vi "Plotmatrix Constructor.vi"(8 "error in (no error)":errorcluster, 9 "y matrix":dbl[][](array[numeric]), 10 "x matrix":dbl[][](array[numeric]), 11 "2D Plotmatrix Datatype.lvclass in":refnum<class "XY Plot Matrix Datatype.lvclass">) -> (0 "error out":errorcluster, 3 "2D Plotmatrix Datatype.lvclass out":refnum<class "XY Plot Matrix Datatype.lvclass">)   [LabVIEW 2020, in "XY Plot Matrix Datatype.lvclass"]
uses:
  <vilib>/Math Plots/2D Math Plots/XY Plot Matrix/XY Plot Matrix Datatype/XY Plot Matrix Datatype.lvclass
  <vilib>/Math Plots/2D Math Plots/XY Plot Matrix/XY Plot Matrix Datatype/XY Plot Matrix Datatype.lvclass/XY Plot Matrix Datatype.ctl
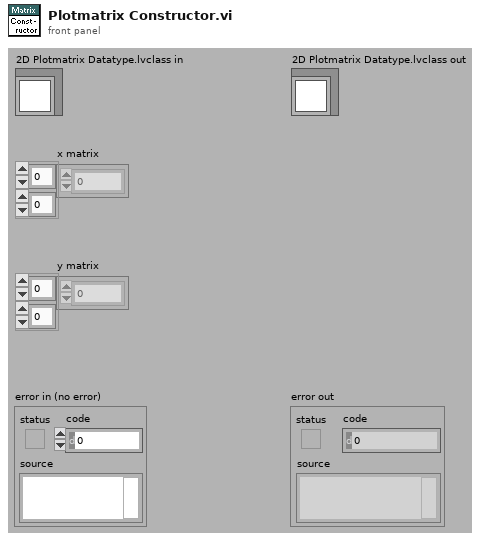
[diagram p1: front panel]
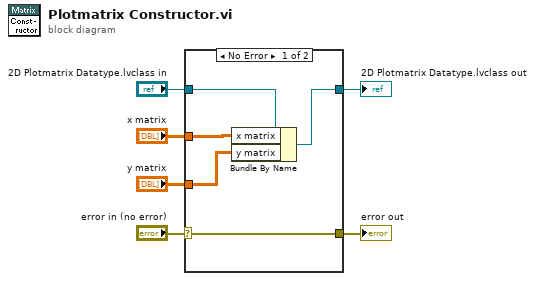
[diagram p0: block diagram]
diagram:
  n1 = case shown="No Error" "error in (no error)" {
    selector: "error in (no error)" -> [w11 w13]
    tunnel: [w11 w13] -> w2
    tunnel: "x matrix" -> [w9 _]
    tunnel: "y matrix" -> [w8 _]
    tunnel: "2D Plotmatrix Datatype.lvclass in" -> [w10 w12]
    tunnel: [w7 w12] -> w6
    frame No Error {
      n2 = Bundle By Name(cluster=w10, "x matrix"=w9, "y matrix"=w8) -> (w7:refnum<class "XY Plot Matrix Datatype.lvclass">)
    }
    frame Error {
    }
  }
  "error out" <- w2
  "2D Plotmatrix Datatype.lvclass out" <- w6
